vi "UI Main.vi"() -> ()   [LabVIEW 2017]
uses:
  Controls/Manual Control.ctl
  Controls/TC Indicator Cluster.ctl
  Controls/LC Calibration Cluster.ctl
  Controls/PS Calibration Cluster.ctl
  Controls/PS Indicator Cluster.ctl
  Controls/Logging Settings.ctl
  Controls/LC Indicator Cluster.ctl
  Support Vis/HOST/cRIO Convert Thermocouple Readings.llb/Thermocouple Type.ctl
  Controls/UI Refs.ctl
  Support Vis/Message Queue/Message Cluster.ctl
  Globals/Host/Global - UI Loop Running.vi
  Globals/Host/Global - UI Streams and Variables.vi
  Globals/Host/Global - Configuration Options.vi
  Support Vis/User Event - Stop/User Event - Stop.lvlib
  Support Vis/Message Queue/Message Queue.lvlib
panel:
  in  "Actuator Settings":T1={"Actuator Settings"=[{"Actuator Name"="IGN O2", "Unpowered State"=0, "Output Port"=1, "Emergency State"=0, "Blank Button"=FALSE, "Open Time [ms]"=0, "Close Time [ms]"=1000}, {"Actuator Name"="IGN H2", "Unpowered State"=0, "Output Port"=2, "Emergency State"=0, "Blank Button"=FALSE, "Open Time [ms]"=0, "Close Time [ms]"=0}, {"Actuator Name"="IGN Spark", "Unpowered State"=0, "Output Port"=3, "Emergency State"=1, "Blank Button"=FALSE, "Open Time [ms]"=0, "Close Time [ms]"=0}, {"Actuator Name"="IGN Purge", "Unpowered State"=0, "Output Port"=4, "Emergency State"=0, "Blank Button"=FALSE, "Open Time [ms]"=0, "Close Time [ms]"=0}]} {"Actuator Settings"."Emergency State" items=["Closed", "Open"]; "Actuator Settings"."Output Port" items=["DIDO/DO0", "DIDO/DO1", "DIDO/DO2", "DIDO/DO3", "DIDO/DO4", "DIDO/DO5", "DIDO/DO6", "DIDO/DO7", "DIDO/DO8", "DIDO/DO9", "DIDO/DO10", "DIDO/DO11", "DIDO/DO12", "DIDO/DO13", "DIDO/DO14", "DIDO/DO15", "PWM/DO0", "PWM/DO1", "PWM/DO2", "PWM/DO3", "PWM/DO4", "PWM/DO5", "PWM/DO6", "PWM/DO7"]; "Actuator Settings"."Unpowered State" items=["Closed", "Opened"]}
  in  "Clear":bool
  out "Logging State":T2(ring)
  out "FPGA States":T3(ring)
  in  "EMERGENCY":bool
  out "Connected?":bool
  in  "Connect to Controller":bool
  in  "Controller Address":string="169.254.173.87"
  out "System Status":string
  in  "Settings Tab":T4(tab)
  in  "Thermocouple types":T5[](array[typedef])=[3, 3, 3, 3, 3, 3, 3, 3, 3, 3, 6, 6, 6, 6, 6, 6] items=["B", "E", "J", "K", "R", "S", "T", "N"]
  in  "PS Calibration":T6
  in  "LC Calibration":T7
  out "Ready to log":bool
  in  "Folder Name":string
  in  "Close File":bool
  in  "Create File":bool
  in  "Clear File History":bool
  out "Logging":bool
  out "Logging File History (Current Session)":string
  in  "Toggle Logging Mode":bool
  out "High Speed":bool
  out "Low Speed":bool
  in  "Stop Logging":bool
  in  "Start Logging":bool
  in  "Logging File Name":string
  in  "Logging Settings":T8
  in  "Toggle Manual Mode":bool
  out "Manual Mode":bool
  out "Ready":bool
  in  "Start AC":bool
  out "Test Timer":dbl
  out "LC Data Cluster":T9 {"LC 4" scale=0.0..10.0; "LC 3" scale=0.0..10.0; "LC 2" scale=0.0..10.0; "LC 1" scale=0.0..10.0}
  out "TC Cluster":T10 {"TC 16" scale=0.0..100.0; "TC 15" scale=0.0..100.0; "TC 14" scale=0.0..100.0; "TC 13" scale=0.0..100.0; "TC 12" scale=0.0..100.0; "TC 11" scale=0.0..100.0; "TC 10" scale=0.0..100.0; "TC 9" scale=0.0..100.0; "TC 8" scale=0.0..100.0; "TC 7" scale=0.0..100.0; "TC 6" scale=0.0..100.0; "TC 5" scale=0.0..100.0; "TC 4" scale=0.0..100.0; "TC 3" scale=0.0..100.0; "TC 2" scale=0.0..100.0; "TC 1" scale=0.0..2.0}
  out "PS Indicator Cluster":T11 {"PS 6" scale=0.0..5.0 scale format="%#.2f"; "PS 5" scale=0.0..5.0 scale format="%#.2f"; "PS 4" scale=0.0..5.0 scale format="%#.2f"; "PS 3" scale=0.0..5.0 scale format="%#.2f"; "PS 2" scale=0.0..5.0 scale format="%#.2f"; "PS 1" scale=0.0..5.0 scale format="%#.2f"}
  out "TC Sensor Chart":T12(graph)
  out "LC Sensor Chart":T13(graph)
  out "PS Sensor Chart":T14(graph)
  in  "Open TDMS Viewer":bool
  in  "Open File Downloader":bool
  # "DARE RIO Test Software"
  # "Name                                      Unpowered State          Output Port                   Emergency State          Manual Control    Open Time[ms]  Close Time[ms]"
  # "Connection Settings"
  # "Pressure Sensors"
  # "Logging Settings"
  # "Logging settings apply when crearting a new file"
  # "Logging File Creation"
  # "Logging"
  # "Automated Sequence Timer"
  # "Automated Sequence Control"
  # "Pressure Sensors"
  # "Load Sensors"
  # "Temperature Sensors"
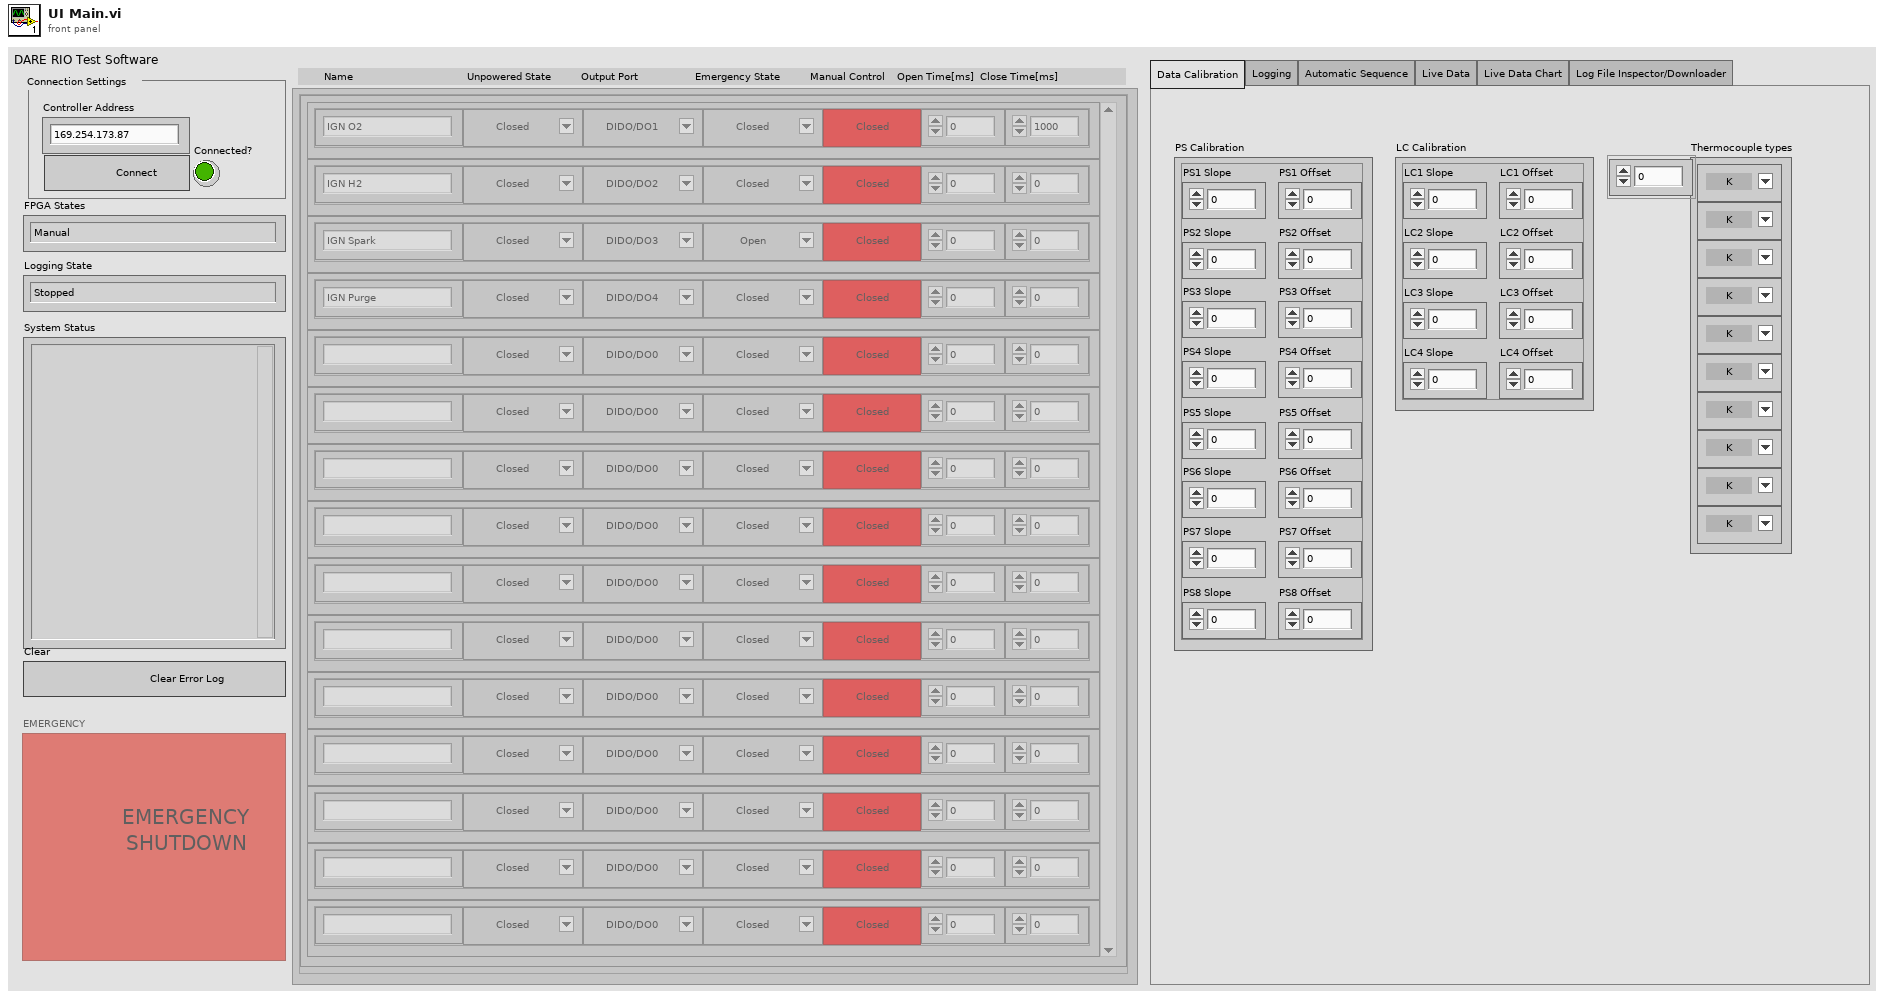
[diagram p1: front panel]
types:
  T1 = typedef "Manual Control.ctl" = cluster{"Actuator Settings":cluster{"Actuator Name":string, "Unpowered State":i16, "Output Port":u32, "Emergency State":i16, "Blank Button":bool, "Open Time [ms]":i16, "Close Time [ms]":i16}[]}
  T2 = enum16{"Stopped", "Logging - Low Speed", "Logging - High Speed"}
  T3 = enum16{"Manual", "Standby", "Automated Sequence", "Automated Sequence End", "Emergency"}
  T4 = enum32{"Data Calibration", "Logging", "Automatic Sequence", "Live Data", "Live Data Chart", "Log File Inspector/Downloader"}
  T5 = typedef "Thermocouple Type.ctl" = u16
  T6 = typedef "PS Calibration Cluster.ctl" = cluster{"PS1 Slope":dbl, "PS1 Offset":dbl, "PS2 Slope":dbl, "PS2 Offset":dbl, "PS3 Slope":dbl, "PS3 Offset":dbl, "PS4 Slope":dbl, "PS4 Offset":dbl, "PS5 Slope":dbl, "PS5 Offset":dbl, "PS6 Slope":dbl, "PS6 Offset":dbl, "PS7 Slope":dbl, "PS7 Offset":dbl, "PS8 Slope":dbl, "PS8 Offset":dbl}
  T7 = typedef "LC Calibration Cluster.ctl" = cluster{"LC1 Slope":dbl, "LC1 Offset":dbl, "LC2 Slope":dbl, "LC2 Offset":dbl, "LC3 Slope":dbl, "LC3 Offset":dbl, "LC4 Slope":dbl, "LC4 Offset":dbl}
  T8 = typedef "Logging Settings.ctl" = cluster{"Logging Channels":cluster{"TC Logging":cluster{"TC 0":bool, "TC 1":bool, "TC 2":bool, "TC 3":bool, "TC 4":bool, "TC 5":bool, "TC 6":bool, "TC 7":bool, "TC 8":bool, "TC 9":bool, "TC 10":bool, "TC 11":bool, "TC 12":bool, "TC 13":bool, "TC 14":bool, "TC 15":bool}, "PS Logging":cluster{"PS 0":bool, "PS 1":bool, "PS 2":bool, "PS 3":bool, "PS 4":bool, "PS 5":bool, "PS 6":bool, "PS 7":bool}, "LC Logging":cluster{"LC 0":bool, "LC 1":bool, "LC 2":bool, "LC 3":bool}}, "TC Low Speed Logging [Hz]":u32, "TC High Speed Logging [Hz]":u32, "PS Low Speed Logging [Hz]":u32, "PS High Speed Logging [Hz]":u32, "LC Low Speed Logging [Hz]":u32, "LC High Speed Logging[Hz]":u32, "Valve Names":string[]}
  T9 = typedef "LC Indicator Cluster.ctl" = cluster{"LC 1":dbl, "LC 2":dbl, "LC 3":dbl, "LC 4":dbl}
  T10 = typedef "TC Indicator Cluster.ctl" = cluster{"TC 1":dbl, "TC 2":dbl, "TC 3":dbl, "TC 4":dbl, "TC 5":dbl, "TC 6":dbl, "TC 7":dbl, "TC 8":dbl, "TC 9":dbl, "TC 10":dbl, "TC 11":dbl, "TC 12":dbl, "TC 13":dbl, "TC 14":dbl, "TC 15":dbl, "TC 16":dbl}
  T11 = typedef "PS Indicator Cluster.ctl" = cluster{"PS 1":dbl, "PS 2":dbl, "PS 3":dbl, "PS 4":dbl, "PS 5":dbl, "PS 6":dbl}
  T12 = cluster{"TC 1":dbl, "TC 2":dbl, "TC 3":dbl, "TC 4":dbl, "TC 5":dbl, "TC 6":dbl, "TC 7":dbl, "TC 8":dbl, "TC 9":dbl, "TC 10":dbl, "TC 11":dbl, "TC 12":dbl, "TC 13":dbl, "TC 14":dbl, "TC 15":dbl, "TC 16":dbl}
  T13 = cluster{"LC 1":dbl, "LC 2":dbl, "LC 3":dbl, "LC 4":dbl}
  T14 = cluster{"PS 1":dbl, "PS 2":dbl, "PS 3":dbl, "PS 4":dbl, "PS 5":dbl, "PS 6":dbl}
  T15 = typedef "UI Refs.ctl" = cluster{"Manual Mode Toggle":refnum<vi>, "Start AC":refnum<vi>, "Start Logging":refnum<vi>, "Stop Logging":refnum<vi>, "Toggle Logging Speed":refnum<vi>, "Emergency Shutdown":refnum<vi>, "Create Log File":refnum<vi>, "Close Log File":refnum<vi>, "Actuator Controls":refnum<vi>, "Logging Settings":refnum<vi>}
  T16 = typedef "Message Queue.lvlib/All Host Message Queues.ctl" = cluster{"UI":refnum<queue>}
  T17 = enum8{"Enabled", "Disabled", "Disabled and Grayed Out"}
  T18 = typedef "Message Queue.lvlib/Message Cluster.ctl" = cluster{"Message":string, "Message Data":variant}
  T19 = typedef "Variable References.ctl" = cluster{"CPU Usage":refnum<k21>, "Buffer Backlog":refnum<k21>, "Contiguous Memory":refnum<k21>, "Drive Space":refnum<k21>, "Actual Loop Period":refnum<k21>, "LC Data":refnum<k21>, "PS Data":refnum<k21>, "TC Data":refnum<k21>, "Valve States":refnum<k21>, "AC Timer":refnum<k21>}
  T20 = cluster{"Actuator Name":string, "Unpowered State":i16, "Output Port":u32, "Emergency State":i16, "Blank Button":bool, "Open Time [ms]":i16, "Close Time [ms]":i16}[]
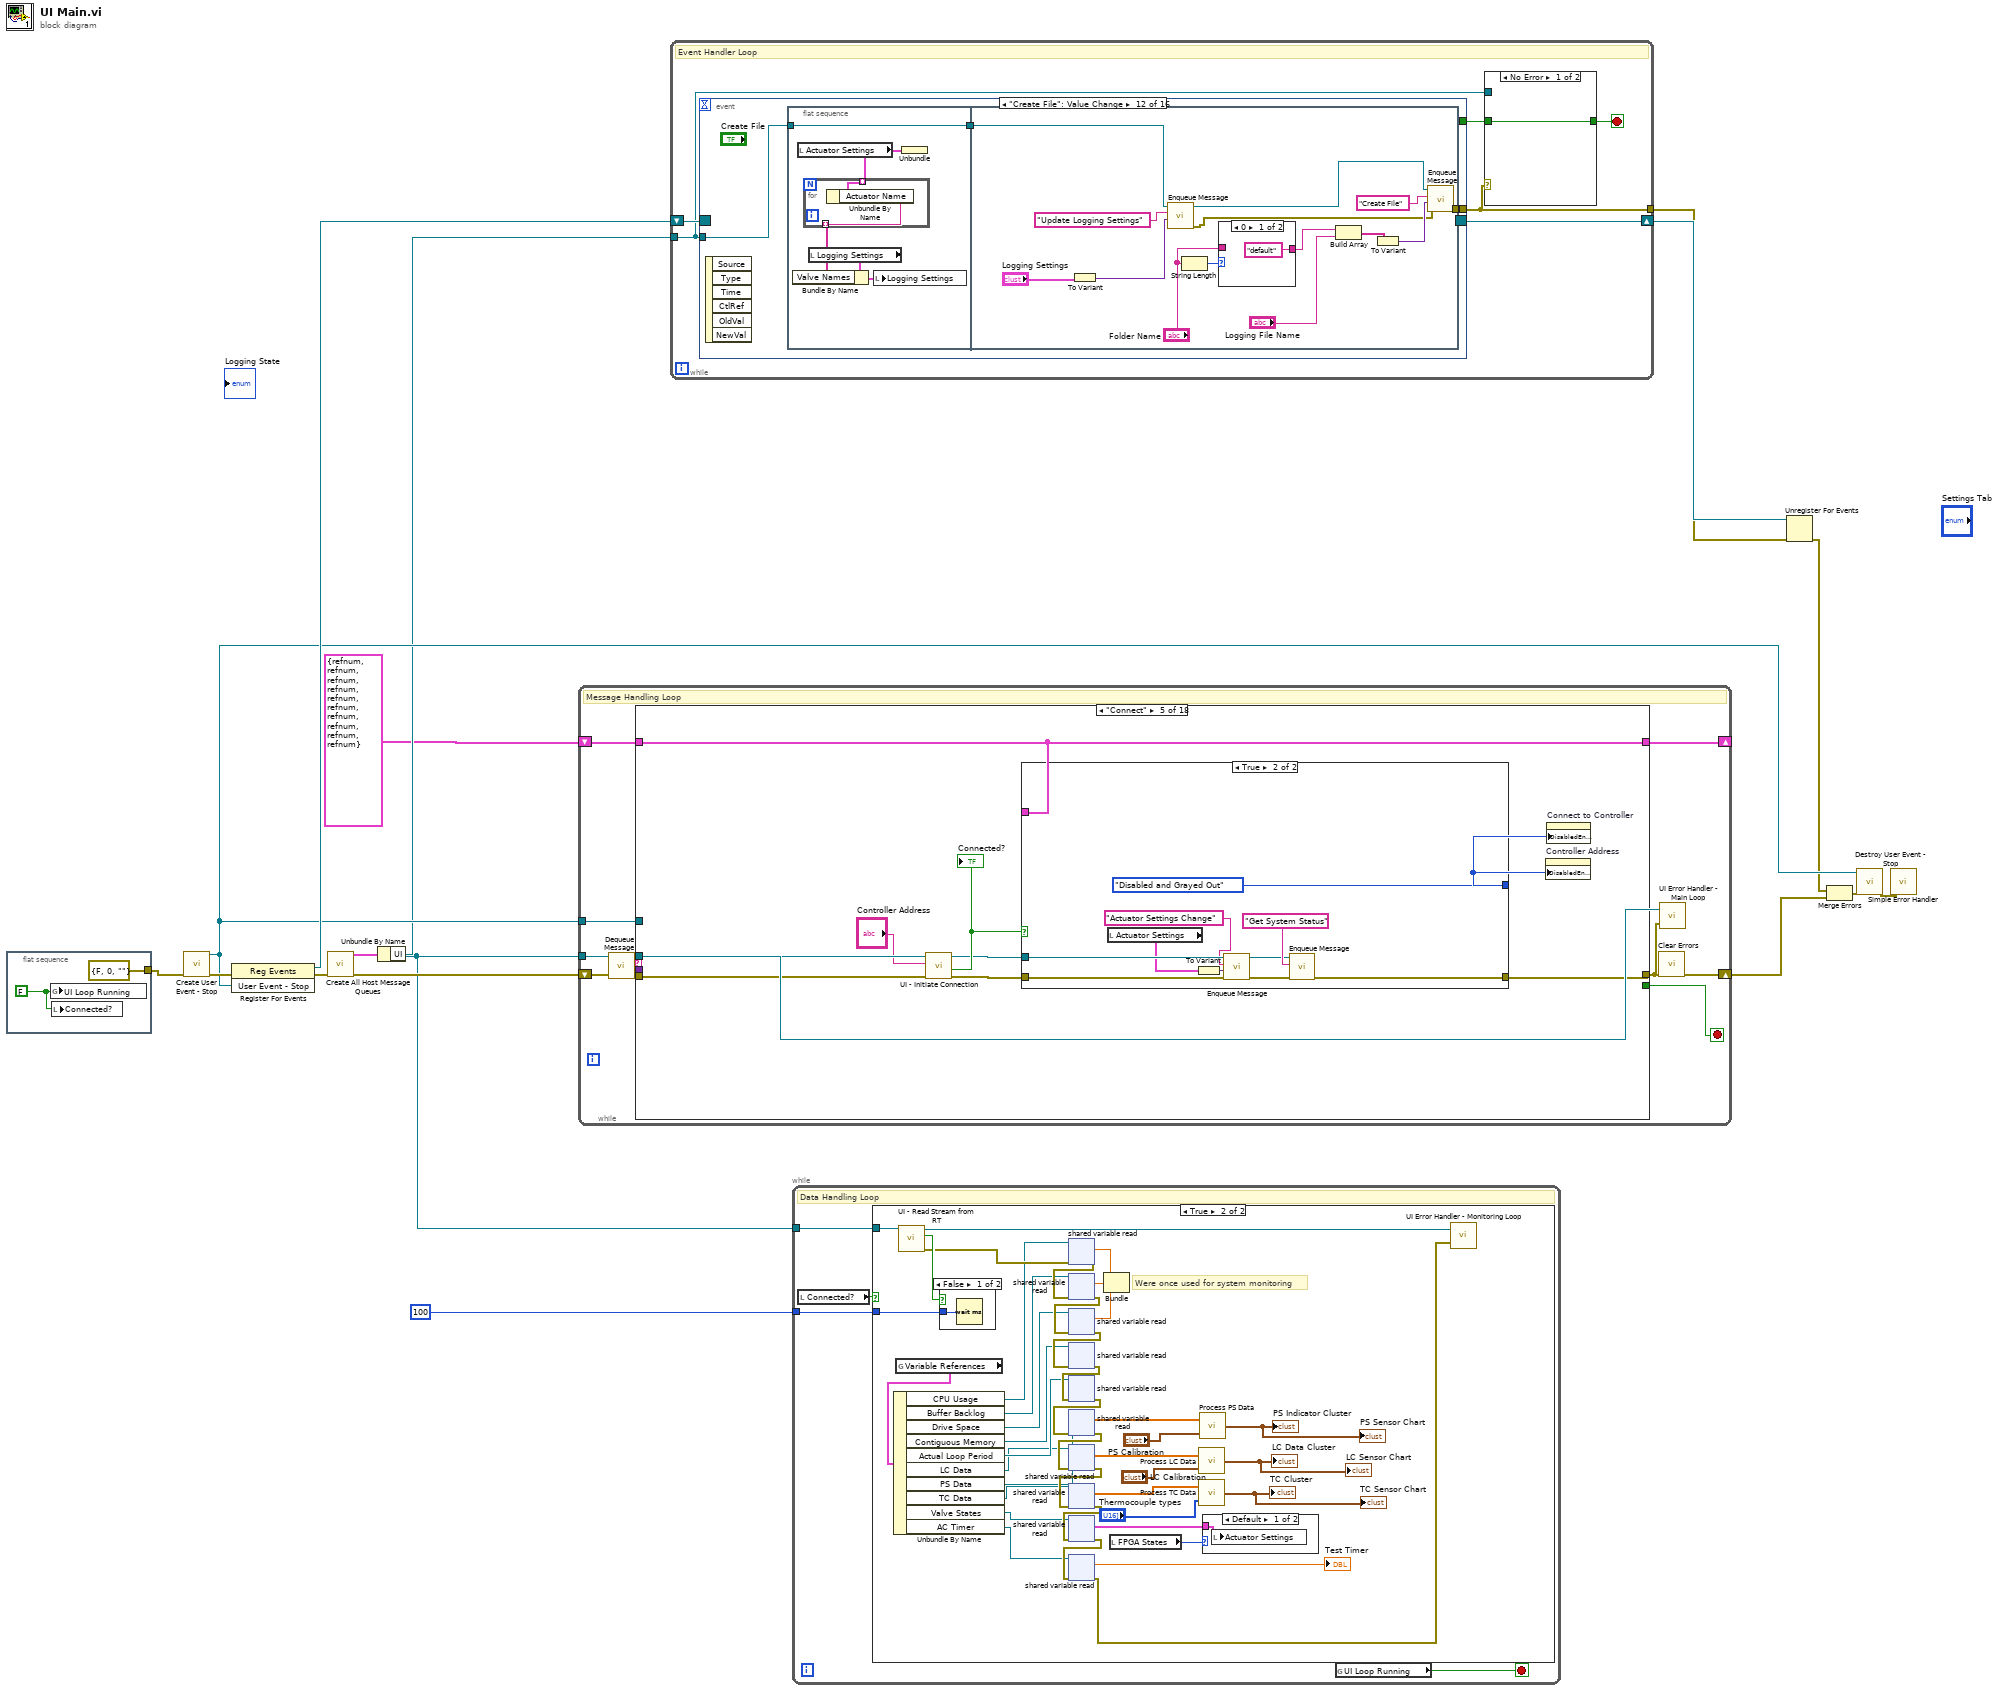
[diagram p0: block diagram]
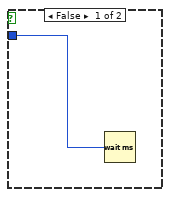
[diagram p2: hidden frame]
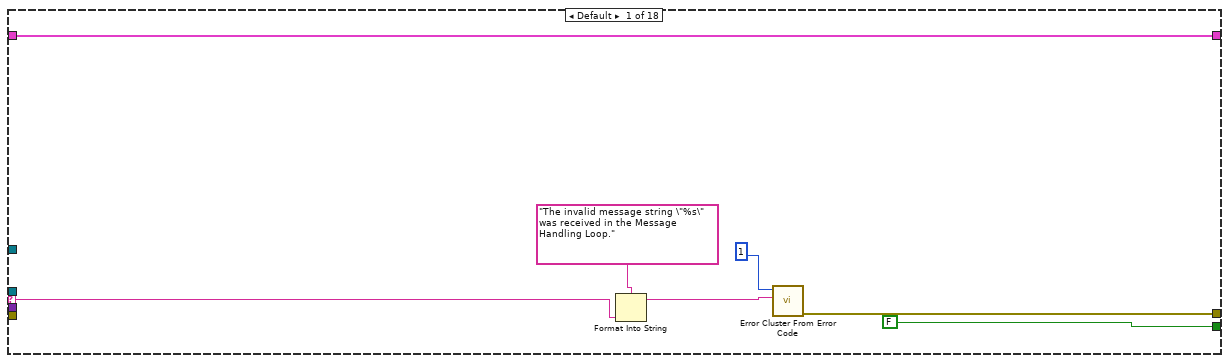
[diagram p5: hidden frame]
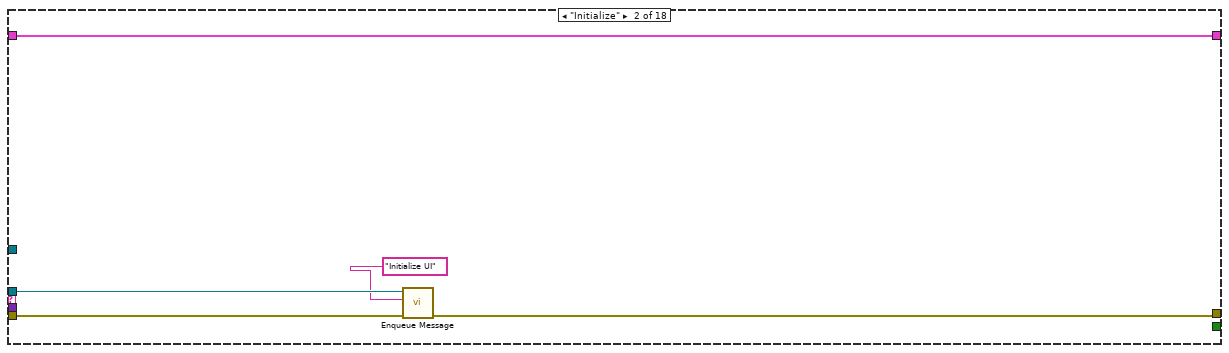
[diagram p6: hidden frame]
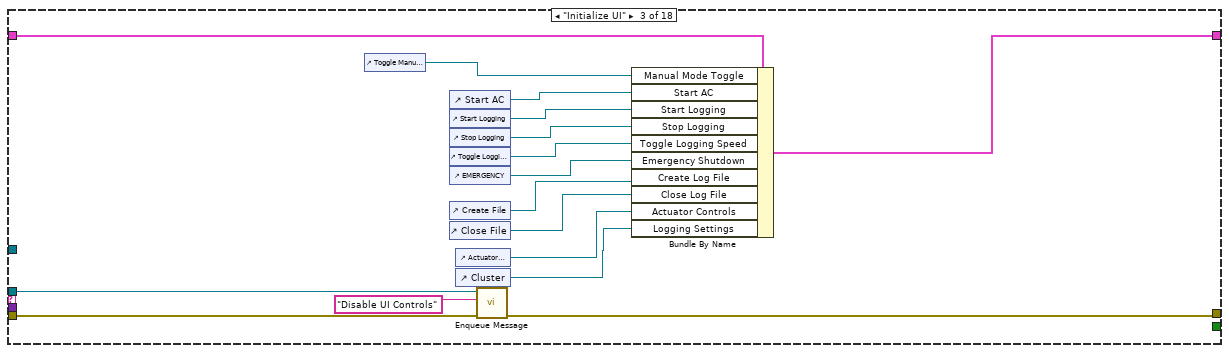
[diagram p7: hidden frame]
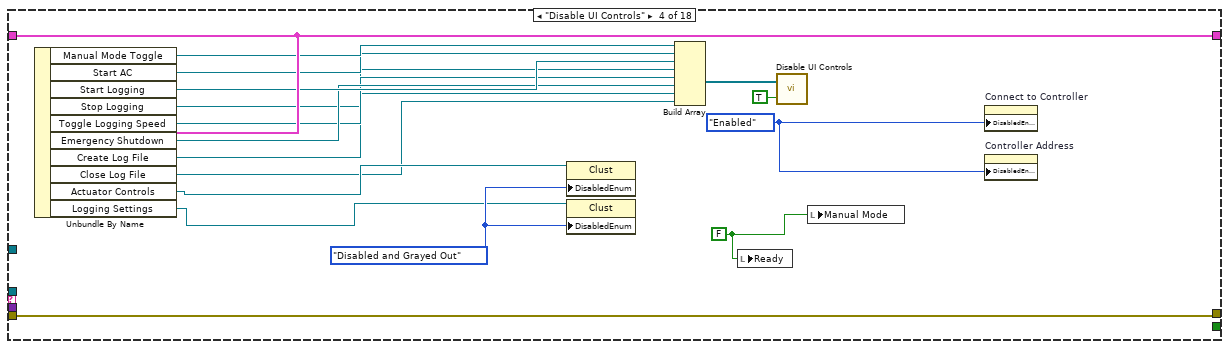
[diagram p8: hidden frame]
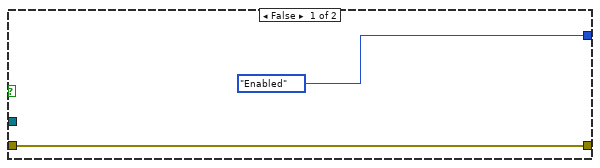
[diagram p9: hidden frame]
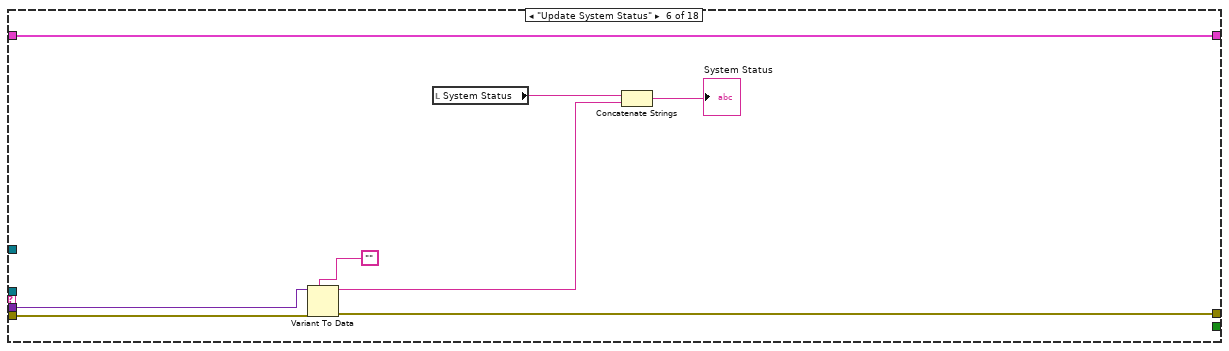
[diagram p10: hidden frame]
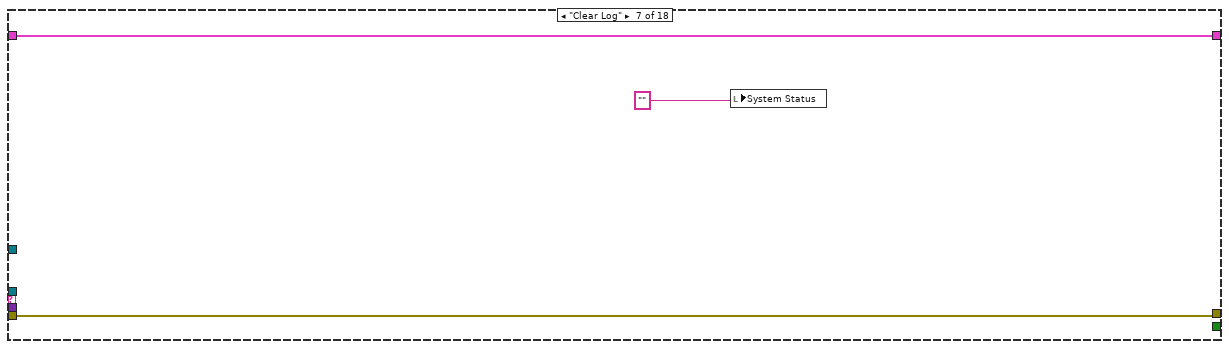
[diagram p11: hidden frame]
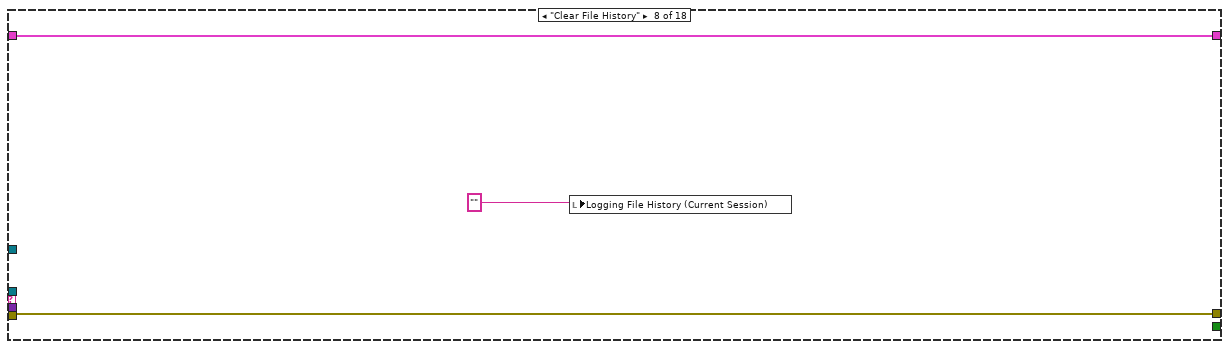
[diagram p12: hidden frame]
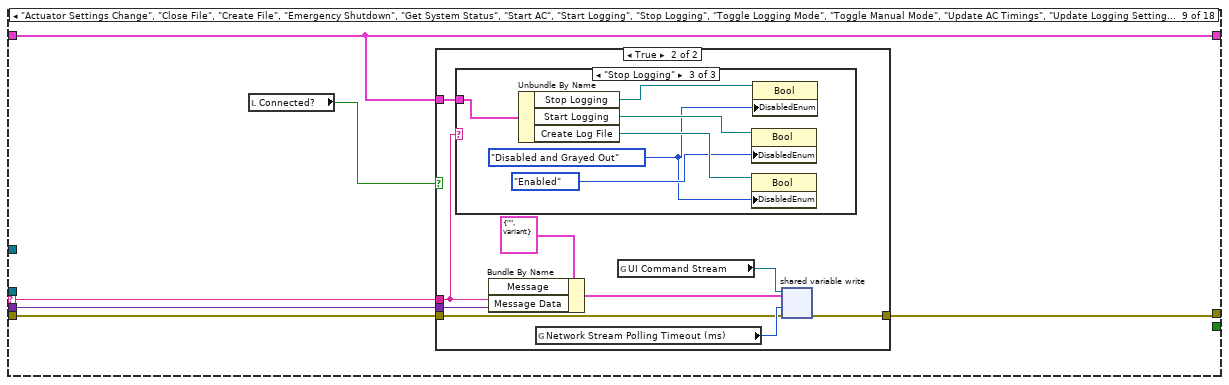
[diagram p13: hidden frame]
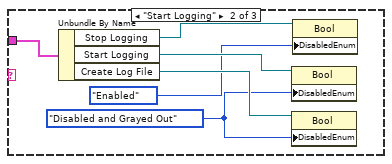
[diagram p16: hidden frame]
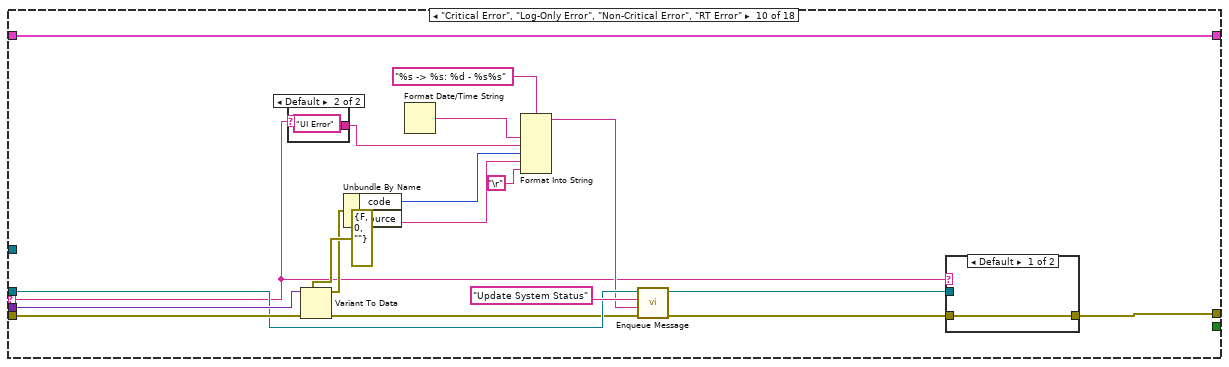
[diagram p17: hidden frame]
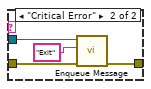
[diagram p18: hidden frame]
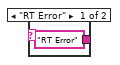
[diagram p19: hidden frame]
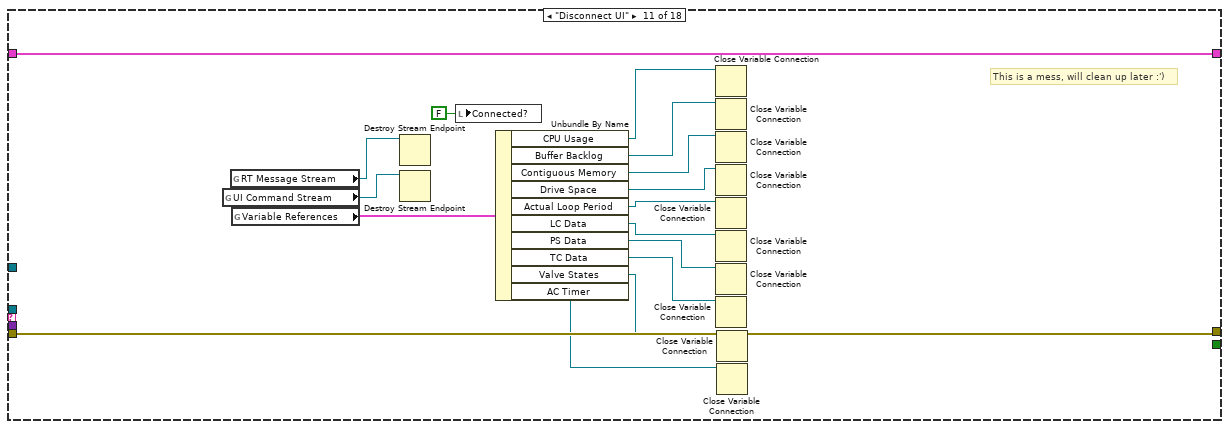
[diagram p20: hidden frame]
diagram:
  n1 = flat-sequence {
    tunnel: [errorcluster {"status"=FALSE, "code"=0, "source"=""} ("error in (no error)")] -> w2
    frame #0 {
      w17 = FALSE
      n2 = global write "Global - UI Loop Running.vi" "UI Loop Running"(w17) -> ()
      n3 = local write "Connected?"(w17) -> ()
    }
  }
  n4 = call "Create User Event - Stop.vi"("error in (no error)"=w2) -> ("error out"=w16:errorcluster, "User Event - Stop"=w9:refnum<user-event>)  [unwired: 9 in]
  n5 = register-events(error in=w16, w9) -> (reference out=w13:refnum<event-registration>, error out=w15:errorcluster)  [unwired: 1 in]
  n6 = call "Create All Host Message Queues.vi"("error in (no error)"=w15) -> ("error out"=w12:errorcluster, "Message Queues out"=w14:T16)  [unwired: 9 in]
  n7 = Unbundle By Name(w14) -> ("UI"=w4:refnum<queue>)
  n8 = while {
    tunnel: w4 -> [w30]
    shift-right: [w26] -> w7
    shift-left: w12 -> [w24]
    tunnel: w9 -> [w21]
    shift-right: [w19] -> _
    shift-left: T15 {"Manual Mode Toggle"=refnum, "Start AC"=refnum, "Start Logging"=refnum, "Stop Logging"=refnum, "Toggle Logging Speed"=refnum, "Emergency Shutdown"=refnum, "Create Log File"=refnum, "Close Log File"=refnum, "Actuator Controls"=refnum, "Logging Settings"=refnum} ("Cluster") -> [w20]
    stop <- w25 stop-if-true
    # "Message Handling Loop"
    n9 = call "Dequeue Message.vi"("error in (no error)"=w24, "Message Queue"=w30) -> ("error out"=w27:errorcluster, "Message Data"=w28:variant, "Message"=w29:string, "dup Message Queue"=w22:refnum<queue>)  [unwired: 6 in]
    n10 = case shown="\"Connect\"" w29 {
      selector: w29 -> [w32 _ _ _ _ _ _ _ w114 w143 _ _ _ _ _ _ _ _]
      tunnel: w22 -> [_ w41 w50 _ w83 _ _ _ _ w146 _ _ _ _ _ _ _ w320]
      tunnel: w28 -> [_ _ _ _ _ w104 _ _ w113 w156 _ _ w188 w198 w248 _ w268 _]
      tunnel: w27 -> [_ w40 w49 w65 w84 w99 w106 w109 w116 w157 w179 w182 w187 w197 w247 w252 w269 w319]
      tunnel: [w33 w39 w47 w65 w78 w98 w106 w109 w115 w140 w179 w182 w186 w195 w246 w252 w265 w313] -> w23
      tunnel: [FALSE _ _ _ _ _ _ _ _ _ _ _ _ _ _ _ _ TRUE] -> w25
      tunnel: w21 -> [_ _ _ _ _ _ _ _ _ _ _ _ _ _ _ _ _ w316]
      tunnel: w20 -> [w31 w42 w58 w75 w77 w97 w105 w110 w112 w139 w178 w181 w189 w194 w241 w257 w266 w312]
      tunnel: [w31 w42 w57 w75 w77 w97 w105 w110 w112 w139 w178 w181 w189 w193 w241 w257 w266 w312] -> w19
      frame Default {
        n11 = Format Into String(format string="The invalid message string \"%s\" was received in the Message Handling Loop." ("Invalid Message Loop Message"), w32) -> (resulting string=w34:string)  [unwired: 2 in, 1 out]
        n12 = call <vilib>:"Error Cluster From Error Code.vi"("error message (\"\")"=w34, "error code (0)"=1) -> ("error out"=w33:errorcluster)  [unwired: 7 in]
      }
      frame "Initialize" {
        n13 = call "Enqueue Message.vi"("error in (no error)"=w40, "Message"="Initialize UI", "Message Queue"=w41) -> ("error out"=w39:errorcluster)  [unwired: 7 in, 1 out]
      }
      frame "Initialize UI" {
        n14 = control-ref of="Toggle Manual Mode"() -> (w46:refnum<vi>)
        n15 = control-ref of="Start AC"() -> (w56:refnum<vi>)
        n16 = control-ref of="Start Logging"() -> (w55:refnum<vi>)
        n17 = control-ref of="Stop Logging"() -> (w54:refnum<vi>)
        n18 = control-ref of="Toggle Logging Mode"() -> (w53:refnum<vi>)
        n19 = control-ref of="EMERGENCY"() -> (w52:refnum<vi>)
        n20 = control-ref of="Create File"() -> (w43:refnum<vi>)
        n21 = control-ref of="Close File"() -> (w44:refnum<vi>)
        n22 = control-ref of="Actuator Settings"() -> (w51:refnum<vi>)
        n23 = control-ref of="Cluster"() -> (w45:refnum<vi>)
        n24 = call "Enqueue Message.vi"("error in (no error)"=w49, "Message"="Disable UI Controls", "Message Queue"=w50) -> ("error out"=w47:errorcluster)  [unwired: 7 in, 1 out]
        n25 = Bundle By Name(cluster=w58, "Manual Mode Toggle"=w46, "Start AC"=w56, "Start Logging"=w55, "Stop Logging"=w54, "Toggle Logging Speed"=w53, "Emergency Shutdown"=w52, "Create Log File"=w43, "Close Log File"=w44, "Actuator Controls"=w51, "Logging Settings"=w45) -> (w57:T15)
      }
      frame "Disable UI Controls" {
        w62 = FALSE ("Manual Mode")
        w63 = T17."Enabled" ("Disabled")
        w64 = T17."Disabled and Grayed Out" ("Disabled")
        n26 = Unbundle By Name(w75) -> ("Manual Mode Toggle"=w74:refnum<vi>, "Start AC"=w70:refnum<vi>, "Start Logging"=w73:refnum<vi>, "Stop Logging"=w69:refnum<vi>, "Toggle Logging Speed"=w71:refnum<vi>, "Emergency Shutdown"=w72:refnum<vi>, "Create Log File"=w68:refnum<vi>, "Close Log File"=w59:refnum<vi>, "Actuator Controls"=w60:refnum<vi>, "Logging Settings"=w61:refnum<vi>)
        n27 = property class="Clust"(reference=w60, "DisabledEnum"=w64) -> ()  [unwired: 1 in, 2 out]
        n28 = property class="Clust"(reference=w61, "DisabledEnum"=w64) -> ()  [unwired: 1 in, 2 out]
        n29 = Build Array(w74, w70, w73, w69, w71, w72, w68, w59) -> (w67:refnum<vi>[])
        n30 = local write "Ready"(w62) -> ()
        n31 = call "Disable UI Controls.vi"("Disable Controls?"=TRUE, "appended array"=w67) -> ()  [unwired: 1 in]
        n32 = local write "Manual Mode"(w62) -> ()
        n33 = property on="Connect to Controller" class="Bool"("DisabledEnum"=w63) -> ()  [unwired: 2 in, 2 out]
        n34 = property on="Controller Address" class="Str"("DisabledEnum"=w63) -> ()  [unwired: 2 in, 2 out]
      }
      frame "Connect" {
        n35 = call "UI - Initiate Connection.vi"("error in (no error)"=w84, "Controller Address"="Controller Address", "Message Queue"=w83) -> ("error out"=w79:errorcluster, "Connected?"=w81:bool, "dup Message Queue"=w80:refnum<queue>)  [unwired: 6 in]
        "Connected?" <- w81
        n36 = case shown="True" w81 {
          tunnel: [T17."Enabled" ("Disabled") T17."Disabled and Grayed Out" ("Disabled")] -> w76
          tunnel: w80 -> [_ w91]
          tunnel: w79 -> [w85 w90]
          tunnel: [w85 w94] -> w78
          tunnel: w77 -> [_ _]
          frame False {
          }
          frame True {
            n37 = local read "Actuator Settings"() -> (w88:T1)
            n38 = To Variant(anything=w88) -> (Variant=w87:variant)
            n39 = call "Enqueue Message.vi"("error in (no error)"=w90, "Message Data"=w87, "Message"="Actuator Settings Change", "Message Queue"=w91) -> ("error out"=w93:errorcluster, "dup Message Queue"=w92:refnum<queue>)  [unwired: 6 in]
            n40 = call "Enqueue Message.vi"("error in (no error)"=w93, "Message"="Get System Status", "Message Queue"=w92) -> ("error out"=w94:errorcluster)  [unwired: 7 in, 1 out]
          }
        }
        n41 = property on="Controller Address" class="Str"("DisabledEnum"=w76) -> ()  [unwired: 2 in, 2 out]
        n42 = property on="Connect to Controller" class="Bool"("DisabledEnum"=w76) -> ()  [unwired: 2 in, 2 out]
      }
      frame "Update System Status" {
        n43 = Variant To Data(error in=w99, type="", Variant=w104) -> (data=w101:string, error out=w98:errorcluster)
        n44 = local read "System Status"() -> (w102:string)
        n45 = Concatenate Strings(w102, w101) -> (→"System Status":string)
      }
      frame "Clear Log" {
        n46 = local write "System Status"("" ("System Status")) -> ()
      }
      frame "Clear File History" {
        n47 = local write "Logging File History (Current Session)"("" ("Logging File History (Current Session)")) -> ()
      }
      frame "Actuator Settings Change", "Close File", "Create File", "Emergency Shutdown", "Get System Status", "Start AC", "Start Logging", "Stop Logging", "Toggle Logging Mode", "Toggle Manual Mode", "Update AC Timings", "Update Logging Settings" {
        n48 = local read "Connected?"() -> (w111:bool)
        n49 = case shown="True" w111 {
          tunnel: w116 -> [w117 w124]
          tunnel: [w117 w126] -> w115
          tunnel: w114 -> [_ w119]
          tunnel: w113 -> [_ w122]
          tunnel: w112 -> [_ w118]
          frame False {
          }
          frame True {
            n50 = case shown="\"Stop Logging\"" w119 {
              tunnel: w118 -> [_ w132 w134]
              frame Default {
              }
              frame "Start Logging" {
                w129 = T17."Disabled and Grayed Out" ("Disabled")
                n51 = Unbundle By Name(w132) -> ("Stop Logging"=w127:refnum<vi>, "Start Logging"=w131:refnum<vi>, "Create Log File"=w130:refnum<vi>)
                n52 = property class="Bool"(reference=w131, "DisabledEnum"=w129) -> ()  [unwired: 1 in, 2 out]
                n53 = property class="Bool"(reference=w130, "DisabledEnum"=w129) -> ()  [unwired: 1 in, 2 out]
                n54 = property class="Bool"(reference=w127, "DisabledEnum"=T17."Enabled" ("Disabled")) -> ()  [unwired: 1 in, 2 out]
              }
              frame "Stop Logging" {
                w133 = T17."Disabled and Grayed Out" ("Disabled")
                n55 = Unbundle By Name(w134) -> ("Stop Logging"=w136:refnum<vi>, "Start Logging"=w138:refnum<vi>, "Create Log File"=w137:refnum<vi>)
                n56 = property class="Bool"(reference=w138, "DisabledEnum"=T17."Enabled" ("Disabled")) -> ()  [unwired: 1 in, 2 out]
                n57 = property class="Bool"(reference=w137, "DisabledEnum"=w133) -> ()  [unwired: 1 in, 2 out]
                n58 = property class="Bool"(reference=w136, "DisabledEnum"=w133) -> ()  [unwired: 1 in, 2 out]
              }
            }
            n59 = Bundle By Name(cluster=T18 {"Message"="", "Message Data"=variant} ("Message Cluster"), "Message"=w119, "Message Data"=w122) -> (w123:T18)
            n60 = global read "Global - Configuration Options.vi" "Network Stream Polling Timeout (ms)"() -> (w125:i32)
            n61 = global read "Global - UI Streams and Variables.vi" "UI Command Stream"() -> (w120:refnum<k21>)
            n62 = shared-variable-write(w120, w124, w123, w125) -> (w126:errorcluster)  [unwired: 2 out]
          }
        }
      }
      frame "Critical Error", "Log-Only Error", "Non-Critical Error", "RT Error" {
        n63 = case shown="Default" w143 {
          tunnel: ["RT Error" "UI Error"] -> w149
          frame "RT Error" {
          }
          frame Default {
          }
        }
        n64 = Variant To Data(error in=w157, type=errorcluster {"status"=FALSE, "code"=0, "source"=""} ("error constant"), Variant=w156) -> (data=w152:errorcluster, error out=w145:errorcluster)
        n65 = Unbundle By Name(w152) -> ("code"=w150:i32, "source"=w151:string)
        n66 = Format Date/Time String() -> (date/time string=w148:string)  [unwired: 3 in]
        n67 = Format Into String(format string="%s -> %s: %d - %s%s", w148, w149, w150, w151, "\r") -> (resulting string=w144:string)  [unwired: 2 in, 1 out]
        n68 = call "Enqueue Message.vi"("error in (no error)"=w145, "Message Data"=w144, "Message"="Update System Status", "Message Queue"=w146) -> ("error out"=w141:errorcluster, "dup Message Queue"=w142:refnum<queue>)  [unwired: 6 in]
        n69 = case shown="Default" w143 {
          tunnel: w142 -> [_ w162]
          tunnel: w141 -> [w158 w161]
          tunnel: [w158 w160] -> w140
          frame Default {
          }
          frame "Critical Error" {
            n70 = call "Enqueue Message.vi"("error in (no error)"=w161, "Message"="Exit", "Message Queue"=w162) -> ("error out"=w160:errorcluster)  [unwired: 7 in, 1 out]
          }
        }
      }
      frame "Disconnect UI" {
        # "This is a mess, will clean up later :')"
        n71 = global read "Global - UI Streams and Variables.vi" "UI Command Stream"() -> (w176:refnum<k21>)
        n72 = global read "Global - UI Streams and Variables.vi" "RT Message Stream"() -> (w177:refnum<k21>)
        n73 = global read "Global - UI Streams and Variables.vi" "Variable References"() -> (w175:T19)
        n74 = Destroy Stream Endpoint(11:w177) -> ()  [unwired: 1 in, 1 out]
        n75 = Destroy Stream Endpoint(11:w176) -> ()  [unwired: 1 in, 1 out]
        n76 = local write "Connected?"(FALSE ("Connected?")) -> ()
        n77 = Unbundle By Name(w175) -> ("CPU Usage"=w174:refnum<k21>, "Buffer Backlog"=w173:refnum<k21>, "Contiguous Memory"=w172:refnum<k21>, "Drive Space"=w171:refnum<k21>, "Actual Loop Period"=w170:refnum<k21>, "LC Data"=w169:refnum<k21>, "PS Data"=w168:refnum<k21>, "TC Data"=w167:refnum<k21>, "Valve States"=w166:refnum<k21>, "AC Timer"=w165:refnum<k21>)
        n78 = Close Variable Connection(11:w174) -> ()  [unwired: 1 in, 1 out]
        n79 = Close Variable Connection(11:w173) -> ()  [unwired: 1 in, 1 out]
        n80 = Close Variable Connection(11:w172) -> ()  [unwired: 1 in, 1 out]
        n81 = Close Variable Connection(11:w171) -> ()  [unwired: 1 in, 1 out]
        n82 = Close Variable Connection(11:w170) -> ()  [unwired: 1 in, 1 out]
        n83 = Close Variable Connection(11:w169) -> ()  [unwired: 1 in, 1 out]
        n84 = Close Variable Connection(11:w168) -> ()  [unwired: 1 in, 1 out]
        n85 = Close Variable Connection(11:w167) -> ()  [unwired: 1 in, 1 out]
        n86 = Close Variable Connection(11:w166) -> ()  [unwired: 1 in, 1 out]
        n87 = Close Variable Connection(11:w165) -> ()  [unwired: 1 in, 1 out]
      }
      frame "--------------" {
      }
      frame "Log Speed Changed" {
        n88 = Variant To Data(error in=w187, type=TRUE, Variant=w188) -> (data=w183:bool, error out=w186:errorcluster)
        "High Speed" <- w183
        n89 = Not(x=w183) -> (.not. x?=→"Low Speed":bool)
      }
      frame "Log Status Change" {
        n90 = Variant To Data(error in=w197, type=cluster{bool, bool} {TRUE, TRUE}, Variant=w198) -> (data=w196:cluster{bool, bool}, error out=w195:errorcluster)
        n91 = Unbundle(w196) -> (w191:bool, w190:bool)
        n92 = case shown="False" w191 {
          tunnel: w194 -> [w205 w224]
          tunnel: [w205 w224] -> w193
          tunnel: w190 -> [w201 _]
          frame False {
            n93 = Unbundle By Name(w205) -> ("Start Logging"=w200:refnum<vi>, "Toggle Logging Speed"=w210:refnum<vi>, "Create Log File"=w204:refnum<vi>, "Close Log File"=w203:refnum<vi>, "Stop Logging"=w207:refnum<vi>)
            n94 = local write "Logging"(FALSE ("Logging")) -> ()
            n95 = case shown="False" w201 {
              tunnel: w204 -> [w214 w218]
              tunnel: w203 -> [w213 w219]
              tunnel: [w217 w222] -> w202
              tunnel: w200 -> [w215 w220]
              tunnel: [w216 w221] -> w199
              frame False {
                n96 = Build Array(w213, w215) -> (w216:refnum<vi>[])
                n97 = Build Array(w214) -> (w217:refnum<vi>[])
              }
              frame True {
                n98 = Build Array(w220, w219) -> (w222:refnum<vi>[])
                n99 = Build Array(w218) -> (w221:refnum<vi>[])
              }
            }
            n100 = Build Array (concatenate)(w210, w202) -> (w212:refnum<vi>[])
            n101 = Build Array (concatenate)(w207, w199) -> (w209:refnum<vi>[])
            n102 = call "Disable UI Controls.vi"("Disable Controls?"=FALSE, "appended array"=w212) -> ()  [unwired: 1 in]
            n103 = call "Disable UI Controls.vi"("Disable Controls?"=TRUE, "appended array"=w209) -> ()  [unwired: 1 in]
          }
          frame True {
            n104 = Unbundle By Name(w224) -> ("Start Logging"=w231:refnum<vi>, "Toggle Logging Speed"=w230:refnum<vi>, "Create Log File"=w229:refnum<vi>, "Close Log File"=w223:refnum<vi>, "Stop Logging"=w226:refnum<vi>)
            n105 = Build Array(w231, w230, w229, w223) -> (w233:refnum<vi>[])
            n106 = Build Array(w226) -> (w228:refnum<vi>[])
            n107 = call "Disable UI Controls.vi"("Disable Controls?"=TRUE, "appended array"=w233) -> ()  [unwired: 1 in]
            n108 = call "Disable UI Controls.vi"("Disable Controls?"=FALSE, "appended array"=w228) -> ()  [unwired: 1 in]
            "Logging" <- TRUE ("Logging")
          }
        }
        n109 = local write "Ready to log"(w190) -> ()
      }
      frame "Log File Created" {
        n110 = Unbundle By Name(w241) -> ("Create Log File"=w239:refnum<vi>, "Close Log File"=w235:refnum<vi>)
        n111 = Build Array(w239) -> (w238:refnum<vi>[])
        n112 = Build Array(w235) -> (w236:refnum<vi>[])
        n113 = call "Disable UI Controls.vi"("Disable Controls?"=FALSE, "appended array"=w236) -> ()  [unwired: 1 in]
        n114 = Variant To Data(error in=w247, type=path "" ("path"), Variant=w248) -> (data=w242:path, error out=w246:errorcluster)
        n115 = call "Disable UI Controls.vi"("Disable Controls?"=TRUE, "appended array"=w238) -> ()  [unwired: 1 in]
        n116 = local read "Logging File History (Current Session)"() -> (w250:string)
        n117 = Path To String(path=w242) -> (string=w243:string)
        n118 = Concatenate Strings(w250, w243, "\r") -> (→"Logging File History (Current Session)":string)
        "Ready to log" <- TRUE ("Ready to log")
      }
      frame "Log File Closed" {
        n119 = Unbundle By Name(w257) -> ("Create Log File"=w262:refnum<vi>, "Close Log File"=w258:refnum<vi>, "Start Logging"=w254:refnum<vi>, "Stop Logging"=w255:refnum<vi>, "Toggle Logging Speed"=w256:refnum<vi>)
        n120 = local write "Logging"(FALSE ("Logging")) -> ()
        n121 = local write "Ready to log"(FALSE ("Ready to log")) -> ()
        n122 = Build Array(w262) -> (w261:refnum<vi>[])
        n123 = Build Array(w258, w254, w255, w256) -> (w259:refnum<vi>[])
        n124 = call "Disable UI Controls.vi"("Disable Controls?"=FALSE, "appended array"=w261) -> ()  [unwired: 1 in]
        n125 = call "Disable UI Controls.vi"("Disable Controls?"=TRUE, "appended array"=w259) -> ()  [unwired: 1 in]
      }
      frame "FPGA State Change" {
        n126 = Variant To Data(error in=w269, type=T3."Manual" ("FPGA States 2"), Variant=w268) -> (data=w264:T3, error out=w265:errorcluster)
        "FPGA States" <- w264
        n127 = case shown="\"Standby\"" w264 {
          tunnel: w266 -> [w282 w294 w303 w306 w309]
          frame "Manual", Default {
            w271 = T17."Enabled" ("Disabled")
            n128 = Unbundle By Name(w282) -> ("Start AC"=w281:refnum<vi>, "Emergency Shutdown"=w274:refnum<vi>, "Manual Mode Toggle"=w273:refnum<vi>, "Actuator Controls"=w275:refnum<vi>, "Logging Settings"=w272:refnum<vi>)
            n129 = local write "Manual Mode"(TRUE ("Manual Mode")) -> ()
            n130 = Build Array(w273) -> (w276:refnum<vi>[])
            n131 = Build Array(w281, w274) -> (w280:refnum<vi>[])
            n132 = call "Disable UI Controls.vi"("Disable Controls?"=TRUE, "appended array"=w280) -> ()  [unwired: 1 in]
            n133 = call "Disable UI Controls.vi"("Disable Controls?"=FALSE, "appended array"=w276) -> ()  [unwired: 1 in]
            n134 = property class="Clust"(reference=w275, "DisabledEnum"=w271) -> ()  [unwired: 1 in, 2 out]
            n135 = property class="Clust"(reference=w272, "DisabledEnum"=w271) -> ()  [unwired: 1 in, 2 out]
            "Ready" <- FALSE ("Ready")
          }
          frame "Standby" {
            w284 = T17."Disabled and Grayed Out" ("Disabled")
            n136 = local write "Manual Mode"(FALSE ("Manual Mode")) -> ()
            n137 = Unbundle By Name(w294) -> ("Start AC"=w292:refnum<vi>, "Manual Mode Toggle"=w286:refnum<vi>, "Emergency Shutdown"=w287:refnum<vi>, "Actuator Controls"=w288:refnum<vi>, "Logging Settings"=w285:refnum<vi>)
            n138 = local write "Ready"(TRUE ("Ready")) -> ()
            n139 = Build Array(w287) -> (w289:refnum<vi>[])
            n140 = Build Array(w292, w286) -> (w293:refnum<vi>[])
            n141 = property class="Clust"(reference=w288, "DisabledEnum"=w284) -> ()  [unwired: 1 in, 2 out]
            n142 = property class="Clust"(reference=w285, "DisabledEnum"=w284) -> ()  [unwired: 1 in, 2 out]
            n143 = call "Disable UI Controls.vi"("Disable Controls?"=FALSE, "appended array"=w293) -> ()  [unwired: 1 in]
            n144 = call "Disable UI Controls.vi"("Disable Controls?"=TRUE, "appended array"=w289) -> ()  [unwired: 1 in]
          }
          frame "Automated Sequence" {
            n145 = Unbundle By Name(w303) -> ("Start AC"=w298:refnum<vi>, "Manual Mode Toggle"=w297:refnum<vi>, "Emergency Shutdown"=w296:refnum<vi>)
            n146 = Build Array(w296) -> (w299:refnum<vi>[])
            n147 = Build Array(w298, w297) -> (w302:refnum<vi>[])
            n148 = call "Disable UI Controls.vi"("Disable Controls?"=FALSE, "appended array"=w299) -> ()  [unwired: 1 in]
            n149 = call "Disable UI Controls.vi"("Disable Controls?"=TRUE, "appended array"=w302) -> ()  [unwired: 1 in]
          }
          frame "Automated Sequence End" {
            (unwired) TRUE ("Disable Controls?")
            n150 = Unbundle By Name(w306) -> ("Emergency Shutdown"=w304:refnum<vi>)
            n151 = Build Array(w304) -> (w305:refnum<vi>[])
            n152 = call "Disable UI Controls.vi"("appended array"=w305) -> ()  [unwired: 2 in]
          }
          frame "Emergency" {
            (unwired) FALSE ("Disable Controls?")
            (unwired) TRUE ("Disable Controls?")
            n153 = Unbundle By Name(w309) -> ("Emergency Shutdown"=w310:refnum<vi>, "Manual Mode Toggle"=w307:refnum<vi>)
            n154 = Build Array(w310) -> (w311:refnum<vi>[])
            n155 = Build Array(w307) -> (w308:refnum<vi>[])
            n156 = call "Disable UI Controls.vi"("appended array"=w311) -> ()  [unwired: 2 in]
            n157 = call "Disable UI Controls.vi"("appended array"=w308) -> ()  [unwired: 2 in]
          }
        }
      }
      frame "Exit" {
        n158 = Release Queue(queue=w320, error in (no error)=w319) -> (error out=w315:errorcluster)  [unwired: 1 in, 2 out]
        n159 = call "Fire User Event - Stop.vi"("User Event - Stop"=w316) -> ("error out"=w314:errorcluster)  [unwired: 10 in]
        n160 = global write "Global - UI Loop Running.vi" "UI Loop Running"(FALSE ("UI Loop Running")) -> ()
        n161 = Merge Errors(w314, w315) -> (w313:errorcluster)
      }
    }
    n162 = call <vilib>:"Clear Errors.vi"("error in (no error)"=w23) -> ("error out"=w26:errorcluster)  [unwired: 5 in, 1 out]
    n163 = call "UI Error Handler - Main Loop.vi"("Error In"=w23, "Message Queue"=w22) -> ()  [unwired: 1 in]
  }
  n164 = while {
    tunnel: w4 -> [w321]
    shift-right: [w326] -> w11
    shift-left: w13 -> [w325]
    tunnel: [w324] -> w10
    stop <- w323 stop-if-true
    # "Event Handler Loop"
    n165 = event shown="[11] \"Create File\": Value Change" {
      selector: w325 -> [_ _ _ _ _ _ _ _ _ _ _ _ _ _ _ _]
      dyn-events: [_ _ _ _ _ _ _ _ _ _ _ _ _ _ _ _] -> w326
      timeout: _ -> [_ _ _ _ _ _ _ _ _ _ _ _ _ _ _ _]
      tunnel: w321 -> [_ w334 _ w345 w350 w352 _ _ w359 w362 w365 w368 w395 w399 w401 w404]
      tunnel: [_ w332 _ w344 w348 w351 _ _ w358 w361 w364 w369 w394 w398 w400 w403] -> w324
      tunnel: [_ _ TRUE _ _ _ _ _ _ _ _ _ _ _ _ _] -> w322
      event Timeout {
        n166 = event-data() -> ()  [unwired: 1 in, 3 out]
      }
      event "Connect to Controller": Value Change {
        n167 = event-data() -> ()  [unwired: 1 in, 1 out]
        n168 = call "Enqueue Message.vi"("Message"="Connect", "Message Queue"=w334) -> ("error out"=w332:errorcluster)  [unwired: 8 in, 1 out]
      }
      event User Event {
        n169 = event-data() -> ()  [unwired: 1 in, 4 out]
      }
      event Value Change {
        n170 = event-data() -> ()  [unwired: 1 in, 6 out]
        n171 = local read "Actuator Settings"() -> (w340:T1)
        n172 = Unbundle(w340) -> ("Actuator Settings"=w339:T20)
        n173 = for {
          tunnel: w339 -> [w347] mode=indexing
          tunnel: [w346] -> w337 mode=indexing
          n174 = Unbundle By Name(w347) -> ("Actuator Name"=w346:string)
        }
        n175 = local read "Logging Settings"() -> (w338:T8)
        n176 = Bundle By Name(cluster=w338, "Valve Names"=w337) -> (w336:T8)
        n177 = local write "Logging Settings"(w336) -> ()
        n178 = To Variant(anything="Actuator Settings") -> (Variant=w341:variant)
        n179 = call "Enqueue Message.vi"("Message Data"=w341, "Message"="Actuator Settings Change", "Message Queue"=w345) -> ("error out"=w344:errorcluster)  [unwired: 7 in, 1 out]
      }
      event "Toggle Manual Mode": Value Change {
        n180 = event-data() -> ()  [unwired: 1 in, 6 out]
        n181 = call "Enqueue Message.vi"("Message"="Toggle Manual Mode", "Message Queue"=w350) -> ("error out"=w348:errorcluster)  [unwired: 8 in, 1 out]
      }
      event "Start AC": Value Change {
        n182 = event-data() -> ()  [unwired: 1 in, 6 out]
        n183 = call "Enqueue Message.vi"("Message"="Start AC", "Message Queue"=w352) -> ("error out"=w351:errorcluster)  [unwired: 8 in, 1 out]
      }
      event "Open File Downloader": Value Change {
        n184 = event-data() -> ()  [unwired: 1 in, 6 out]
        n185 = local read "Controller Address"() -> (w354:string)
        n186 = call "File explorer.vi"("IP Address"=w354) -> ()  [unwired: 27 in]
      }
      event "Open TDMS Viewer": Value Change {
        n187 = event-data() -> ()  [unwired: 1 in, 6 out]
        n188 = local read "Thermocouple types"() -> (w355:T5[])
        n189 = local read "LC Calibration"() -> (w356:T7)
        n190 = local read "PS Calibration"() -> (w357:T6)
        n191 = call "Log File Inspector.vi"("Thermocouple types"=w355, "LC Calibration"=w356, "PS Calibration"=w357) -> ()  [unwired: 1 in]
      }
      event "Start Logging": Value Change {
        n192 = event-data() -> ()  [unwired: 1 in, 6 out]
        n193 = call "Enqueue Message.vi"("Message"="Start Logging", "Message Queue"=w359) -> ("error out"=w358:errorcluster)  [unwired: 8 in, 1 out]
      }
      event "Stop Logging": Value Change {
        n194 = event-data() -> ()  [unwired: 1 in, 6 out]
        n195 = call "Enqueue Message.vi"("Message"="Stop Logging", "Message Queue"=w362) -> ("error out"=w361:errorcluster)  [unwired: 8 in, 1 out]
      }
      event "Toggle Logging Mode": Value Change {
        n196 = event-data() -> ()  [unwired: 1 in, 6 out]
        n197 = call "Enqueue Message.vi"("Message"="Toggle Logging Mode", "Message Queue"=w365) -> ("error out"=w364:errorcluster)  [unwired: 8 in, 1 out]
      }
      event "Create File": Value Change {
        n198 = event-data() -> ()  [unwired: 1 in, 6 out]
        n199 = flat-sequence {
          tunnel: w368 -> [w375]
          tunnel: [w375] -> w367
          tunnel: [w389] -> w369
          tunnel: w367 -> [w385]
          frame #0 {
            n200 = local read "Actuator Settings"() -> (w374:T1)
            n201 = local read "Logging Settings"() -> (w372:T8)
            n202 = Unbundle(w374) -> ("Actuator Settings"=w373:T20)
            n203 = for {
              tunnel: w373 -> [w377] mode=indexing
              tunnel: [w376] -> w371 mode=indexing
              n204 = Unbundle By Name(w377) -> ("Actuator Name"=w376:string)
            }
            n205 = Bundle By Name(cluster=w372, "Valve Names"=w371) -> (w370:T8)
            n206 = local write "Logging Settings"(w370) -> ()
          }
          frame #1 {
            n207 = To Variant(anything="Logging Settings") -> (Variant=w384:variant)
            n208 = call "Enqueue Message.vi"("Message Data"=w384, "Message"="Update Logging Settings", "Message Queue"=w385) -> ("error out"=w387:errorcluster, "dup Message Queue"=w386:refnum<queue>)  [unwired: 7 in]
            n209 = String Length(string="Folder Name") -> (length=w380:i32)
            n210 = case shown="0" w380 {
              tunnel: "Folder Name" -> [_ w393]
              tunnel: ["default" w393] -> w378
              frame 0 {
              }
              frame 1, Default {
              }
            }
            n211 = Build Array(w378, "Logging File Name") -> (w381:string[])
            n212 = To Variant(anything=w381) -> (Variant=w390:variant)
            n213 = call "Enqueue Message.vi"("error in (no error)"=w387, "Message Data"=w390, "Message"="Create File", "Message Queue"=w386) -> ("error out"=w389:errorcluster)  [unwired: 6 in, 1 out]
          }
        }
      }
      event "Close File": Value Change {
        n214 = event-data() -> ()  [unwired: 1 in, 6 out]
        n215 = call "Enqueue Message.vi"("Message"="Close File", "Message Queue"=w395) -> ("error out"=w394:errorcluster)  [unwired: 8 in, 1 out]
      }
      event "EMERGENCY": Value Change {
        n216 = event-data() -> ()  [unwired: 1 in, 6 out]
        n217 = call "Enqueue Message.vi"("Message"="Emergency Shutdown", "Message Queue"=w399) -> ("error out"=w398:errorcluster)  [unwired: 8 in, 1 out]
      }
      event "Clear": Value Change {
        n218 = event-data() -> ()  [unwired: 1 in, 6 out]
        n219 = call "Enqueue Message.vi"("Message"="Clear Log", "Message Queue"=w401) -> ("error out"=w400:errorcluster)  [unwired: 8 in, 1 out]
      }
      event "Clear File History": Value Change {
        n220 = event-data() -> ()  [unwired: 1 in, 6 out]
        n221 = call "Enqueue Message.vi"("Message"="Clear File History", "Message Queue"=w404) -> ("error out"=w403:errorcluster)  [unwired: 8 in, 1 out]
      }
    }
    n222 = case shown="No Error" w324 {
      tunnel: [w327 TRUE] -> w323
      tunnel: w322 -> [w327 _]
      tunnel: w321 -> [_ w328]
      frame No Error {
      }
      frame Error {
        n223 = call "Enqueue Message.vi"("Priority Message? (F)"=TRUE, "Message"="Exit", "Message Queue"=w328) -> ()  [unwired: 7 in, 2 out]
      }
    }
  }
  n224 = while {
    tunnel: w4 -> [w406]
    tunnel: u32 100 -> [w407]
    stop <- w409 stop-if-true
    # "Data Handling Loop"
    n225 = local read "Connected?"() -> (w408:bool)
    n226 = case shown="True" w408 {
      tunnel: w407 -> [w410 w449]
      tunnel: w406 -> [_ w451]
      frame False {
        n227 = Wait (ms)(milliseconds to wait=w410) -> ()  [unwired: 1 out]
      }
      frame True {
        # "Were once used for system monitoring"
        n228 = global read "Global - UI Streams and Variables.vi" "Variable References"() -> (w444:T19)
        n229 = Unbundle By Name(w444) -> ("CPU Usage"=w443:refnum<k21>, "Buffer Backlog"=w442:refnum<k21>, "Drive Space"=w441:refnum<k21>, "Contiguous Memory"=w440:refnum<k21>, "Actual Loop Period"=w435:refnum<k21>, "LC Data"=w416:refnum<k21>, "PS Data"=w417:refnum<k21>, "TC Data"=w418:refnum<k21>, "Valve States"=w424:refnum<k21>, "AC Timer"=w423:refnum<k21>)
        n230 = call "UI - Read Stream from RT.vi"("Message Queue"=w451) -> ("error out"=w448:errorcluster, "Message Received?"=w450:bool, "dup Message Queue"=w427:refnum<queue>)  [unwired: 8 in]
        n231 = case shown="False" w450 {
          tunnel: w449 -> [w453 _]
          frame False {
            n232 = Wait (ms)(milliseconds to wait=w453) -> ()  [unwired: 1 out]
          }
          frame True {
          }
        }
        n233 = shared-variable-read(w443, w448) -> (w447:errorcluster, w428:dbl)  [unwired: 2 out]
        n234 = shared-variable-read(w442, w447) -> (w446:errorcluster, w430:dbl)  [unwired: 2 out]
        n235 = shared-variable-read(w441, w446) -> (w445:errorcluster, w429:dbl)  [unwired: 2 out]
        n236 = shared-variable-read(w440, w445) -> (w439:errorcluster)  [unwired: 3 out]
        n237 = shared-variable-read(w435, w439) -> (w438:errorcluster)  [unwired: 3 out]
        n238 = shared-variable-read(w417, w438) -> (w437:errorcluster, w432:dbl[])  [unwired: 2 out]
        n239 = shared-variable-read(w416, w437) -> (w436:errorcluster, w434:dbl[])  [unwired: 2 out]
        n240 = shared-variable-read(w418, w436) -> (w426:errorcluster, w415:dbl[])  [unwired: 2 out]
        n241 = shared-variable-read(w424, w426) -> (w425:errorcluster, w420:T1)  [unwired: 2 out]
        n242 = shared-variable-read(w423, w425) -> (w422:errorcluster, →"Test Timer":dbl)  [unwired: 2 out]
        n243 = Bundle("Double"=w428, "Double"=w430, "Double"=w429) -> ()  [unwired: 1 in, 1 out]
        n244 = local read "FPGA States"() -> (w421:T3)
        n245 = call "Process LC Data.vi"("LC Indicator Cluster"="LC Calibration", "Array"=w434) -> ("PS Data Cluster"=→"LC Data Cluster" →"LC Sensor Chart":T9)
        n246 = call "Process TC Data.vi"("Thermocouple types"="Thermocouple types", "TC Data Raw"=w415) -> ("TC Cluster"=→"TC Cluster" →"TC Sensor Chart":T10)
        n247 = call "Process PS Data.vi"("PS Calibration"="PS Calibration", "Array"=w432) -> ("PS Indicator Cluster"=→"PS Indicator Cluster" →"PS Sensor Chart":T11)
        n248 = case shown="Default" w421 {
          tunnel: w420 -> [w452 _]
          frame Default {
            n249 = local write "Actuator Settings"(w452) -> ()
          }
          frame "Manual" {
          }
        }
        n250 = call "UI Error Handler - Monitoring Loop.vi"("Error In"=w422, "Message Queue"=w427) -> ()  [unwired: 1 in]
      }
    }
    n251 = global read "Global - UI Loop Running.vi" "UI Loop Running"() -> (w409:bool)
  }
  n252 = Unregister For Events(event registration refnum=w11, error in=w10) -> (error out=w6:errorcluster)
  n253 = Merge Errors(w6, w7) -> (w8:errorcluster)
  n254 = call "Destroy User Event - Stop.vi"("error in (no error)"=w8, "User Event - Stop"=w9) -> ("error out"=w5:errorcluster)  [unwired: 9 in]
  n255 = call <vilib>:"Simple Error Handler.vi"("error in (no error)"=w5) -> ()  [unwired: 4 in, 5 out]
